vi "Database Refresh Options.vi"(8 "error in (no error)":errorcluster) -> (0 "error out":errorcluster, 1 "Cancelled?":bool, 2 "Refresh Settings":T1)   [LabVIEW 2013]
uses:
  Controls/Refresh Match Settings.ctl
  AIT 664 Custom Device.lvlib
panel:
  in  "Lbl Selection":enum32{"ByName", "By#"}(radio)=enum."By#" caption="How should database labels be matched to imported labels?"
  out "Vertical Stop Button":bool
  in  "CH Selection":enum32{"ByName", "By#"}(radio) caption="How should database channels be matched to imported channels?"
  in  "Cancel":bool
  in  "Go":bool
  # "Information: Parameters will be merged and matched by name"
  # "WARNING: Proceeding with the refresh could possibly update the system definition by adding, deleting, or modifying channel and label settings."
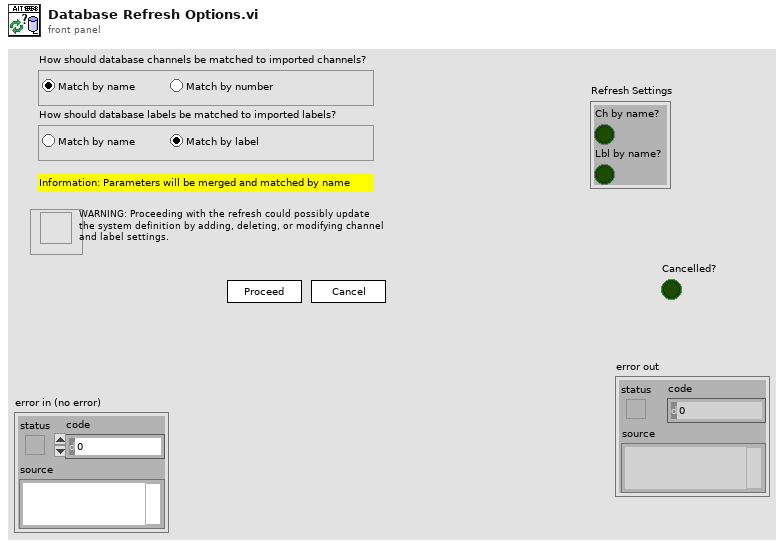
[diagram p1: front panel]
types:
  T1 = typedef "AIT 664 Custom Device.lvlib/Refresh Match Settings.ctl" = cluster{"Ch by name?":bool, "Lbl by name?":bool}
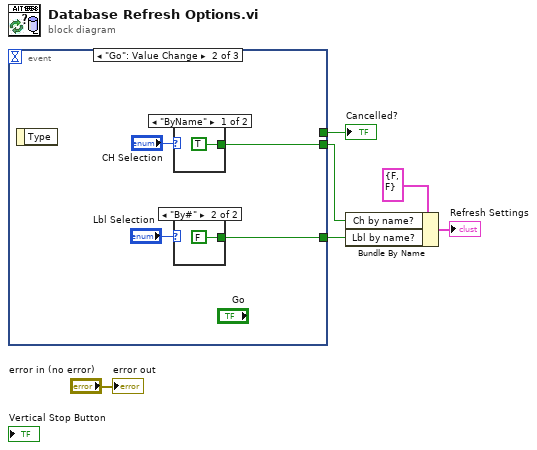
[diagram p0: block diagram]
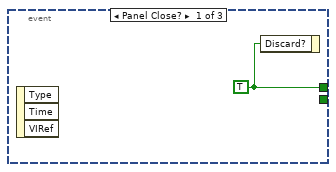
[diagram p2: hidden frame]
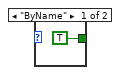
[diagram p3: hidden frame]
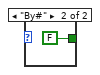
[diagram p4: hidden frame]
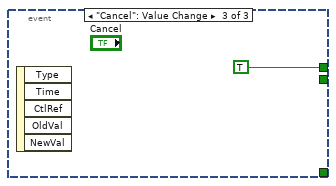
[diagram p5: hidden frame]
diagram:
  n1 = event shown="[1] \"Go\": Value Change" {
    selector: _ -> [_ _ _]
    dyn-events: _ -> [_ _ _]
    timeout: _ -> [_ _ _]
    tunnel: [_ w10 _] -> w2
    tunnel: [w7 _ TRUE ("Discard?")] -> w5
    tunnel: [_ w8 _] -> w1
    event Panel Close? {
      w7 = TRUE ("Discard?")
      n2 = event-data() -> ()  [unwired: 1 in, 3 out]
      n3 = event-data("Discard?"=w7) -> ()  [unwired: 1 in, 1 out]
    }
    event "Go": Value Change {
      n4 = event-data() -> ()  [unwired: 1 in, 1 out]
      n5 = case shown="\"ByName\"" "CH Selection" {
        tunnel: [TRUE ("Match Channels By Name?") FALSE ("Match Channels By Name?")] -> w10
        frame "ByName" {
        }
        frame "By#" {
        }
      }
      n6 = case shown="\"By#\"" "Lbl Selection" {
        tunnel: [TRUE ("Match Channels By Name?") FALSE ("Match Channels By Name?")] -> w8
        frame "ByName" {
        }
        frame "By#" {
        }
      }
    }
    event "Cancel": Value Change {
      n7 = event-data() -> ()  [unwired: 1 in, 5 out]
    }
  }
  "Cancelled?" <- w5
  n8 = Bundle By Name(cluster=T1 {"Ch by name?"=FALSE, "Lbl by name?"=FALSE} ("Refresh Settings"), "Ch by name?"=w2, "Lbl by name?"=w1) -> (→"Refresh Settings":T1)
  "error out" <- "error in (no error)"
